vi "Slide Prevention.vi"(11 "Slide?":bool) -> ()   [LabVIEW 2017]
uses:
  <vilib>/Rock Robotics/WPI/Solenoid/WPI_SolenoidValue.ctl
  <vilib>/Rock Robotics/WPI/Solenoid/WPI_SolenoidSetEnum.vi
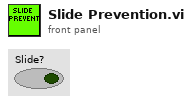
[diagram p1: front panel]
types:
  T1 = typedef "WPI_SolenoidValue.ctl" = enum16{"Off", "On", "Forward", "Reverse"}
  T2 = typedef "WPI_SolenoidDevRef.ctl" = cluster{"DevStatus":errorcluster, "Pneumatics Control Module":u8, "Forward Solenoid Channel":T3, "Reverse Solenoid Channel":T3}
  T3 = typedef "WPI_SolenoidChannel.ctl" = enum8{"Solenoid 0", "Solenoid 1", "Solenoid 2", "Solenoid 3", "Solenoid 4", "Solenoid 5", "Solenoid 6", "Solenoid 7", "Invalid"}
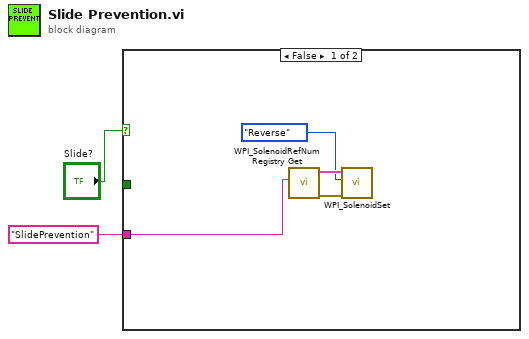
[diagram p0: block diagram]
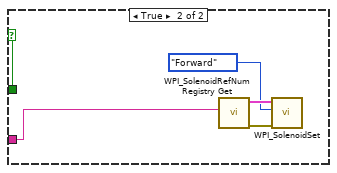
[diagram p2: hidden frame]
diagram:
  n1 = case shown="False" "Slide?" {
    selector: "Slide?" -> [_ w8]
    tunnel: [_ w8] -> _
    tunnel: "SlidePrevention" ("refnum name") -> [w3 w7]
    frame False {
      n2 = call <vilib>:"WPI_SolenoidRefNum Registry Get.vi"("refnum name"=w3) -> ("error out"=w5:errorcluster, "SolenoidDevRef"=w6:T2)  [unwired: 9 in]
      n3 = call-poly <vilib>:"WPI_SolenoidSet.vi"("error in (no error)"=w5, "Value"=WPI_SolenoidValue."Reverse", "SolenoidDevRef"=w6) -> ()  [unwired: 7 in, 2 out]
    }
    frame True {
      n4 = call <vilib>:"WPI_SolenoidRefNum Registry Get.vi"("refnum name"=w7) -> ("error out"=w11:errorcluster, "SolenoidDevRef"=w10:T2)  [unwired: 9 in]
      n5 = call-poly <vilib>:"WPI_SolenoidSet.vi"("error in (no error)"=w11, "Value"=WPI_SolenoidValue."Forward", "SolenoidDevRef"=w10) -> ()  [unwired: 7 in, 2 out]
    }
  }
